vi "Example.vi"() -> ()   [LabVIEW 2019]
uses:
  fd21ea2b-fe82-4c24-8fbe-779a5f18eb94.vi
  193783c4-9c22-43a6-9abe-7ec735545827.vi
  ad1777d4-6ecb-4841-a2c2-9d75e62a62a5.vi
  LV Colormap Names.ctl
panel:
  in  "Stop":bool
  in  "Tab Control":T1(tab)
  in  "Colormap Name (original enum)":T2=enum."turbo"
  in  "Colormap Name (reduced enum)":T3(ring)=enum."inferno"
  in  "Colormap By Name":string="gist_stern"
  in  "Example Data Name":u16(ring)=8 items=["PC Fan"=0, "Noisy Chirps"=1, "TDR 1"=2, "TDR 2"=3, "Liquefaction"=4, "Liquefaction Free"=5, "Aneurysm"=6, "Bat"=7, "RF"=8, "Two Gaussian"=9, "Three Gaussian"=10, "Chirp"=11, "Gaussian Chirp"=12, "Cross Chirp"=13, "Doppler"=14, "HOP"=15, "TF Sine"=16, "Three Tone"=17, "Four Tone"=23, "Blood Flow Doppler (phase a)"=20, "Blood Flow Doppler (phase b)"=21, "Heart sound"=22, "Random Noise"=19]
  out "Signals":waveform(dbl)(graph)={"t0"=timestamp(0 s since 1904-01-01), "dt"=1e-09, "Y"=[]}
  out "Magnitude of Gabor Coefficients":dbl[][](graph)
  # "ex:\nnipy_spectral\ngnuplot\ngist_stern"
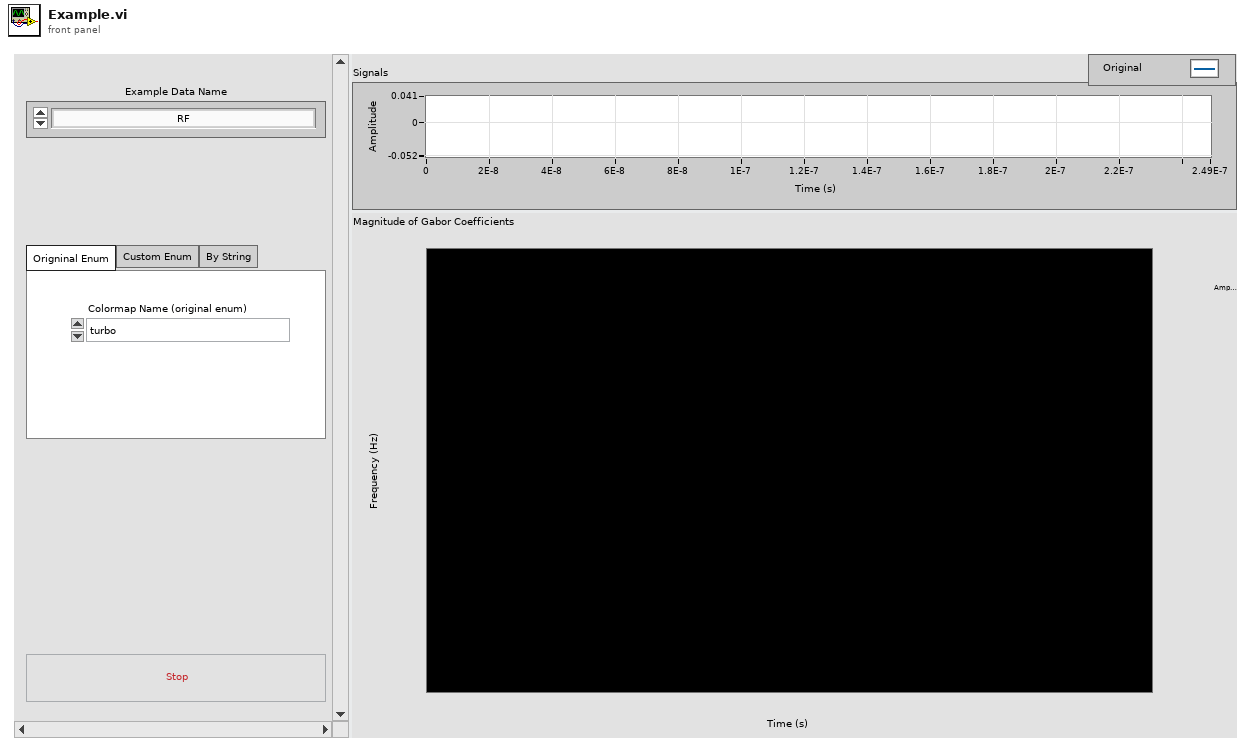
[diagram p1: front panel]
types:
  T1 = enum32{"Origninal Enum", "Custom Enum", "By String"}
  T2 = typedef "LV Colormap Names.ctl" = enum16{"Accent", "Accent_r", "Blues", "Blues_r", "BrBG", "BrBG_r", "BuGn", "BuGn_r", "BuPu", "BuPu_r", "CMRmap", "CMRmap_r", "Dark2", "Dark2_r", "GnBu", "GnBu_r", "Grays", "Grays_r", "Greens", "Greens_r", "Greys", "Greys_r", "OrRd", "OrRd_r", "Oranges", "Oranges_r", "PRGn", "PRGn_r", "Paired", "Paired_r", "Pastel1", "Pastel1_r", "Pastel2", "Pastel2_r", "PiYG", "PiYG_r", "PuBu", "PuBuGn", "PuBuGn_r", "PuBu_r", "PuOr", "PuOr_r", "PuRd", "PuRd_r", "Purples", "Purples_r", "RdBu", "RdBu_r", "RdGy", "RdGy_r", "RdPu", "RdPu_r", "RdYlBu", "RdYlBu_r", "RdYlGn", "RdYlGn_r", "Reds", "Reds_r", "Set1", "Set1_r", "Set2", "Set2_r", "Set3", "Set3_r", "Spectral", "Spectral_r", "Wistia", "Wistia_r", "YlGn", "YlGnBu", "YlGnBu_r", "YlGn_r", "YlOrBr", "YlOrBr_r", "YlOrRd", "YlOrRd_r", "afmhot", "afmhot_r", "autumn", "autumn_r", "berlin", "berlin_r", "binary", "binary_r", "bone", "bone_r", "brg", "brg_r", "bwr", "bwr_r", "cividis", "cividis_r", "cool", "cool_r", "coolwarm", "coolwarm_r", "copper", "copper_r", "cubehelix", "cubehelix_r", "flag", "flag_r", "gist_earth", "gist_earth_r", "gist_gray", "gist_gray_r", "gist_grey", "gist_grey_r", "gist_heat", "gist_heat_r", "gist_ncar", "gist_ncar_r", "gist_rainbow", "gist_rainbow_r", "gist_stern", "gist_stern_r", "gist_yarg", "gist_yarg_r", "gist_yerg", "gist_yerg_r", "gnuplot", "gnuplot2", "gnuplot2_r", "gnuplot_r", "gray", "gray_r", "grey", "grey_r", "hot", "hot_r", "hsv", "hsv_r", "inferno", "inferno_r", "jet", "jet_r", "magma", "magma_r", "managua", "managua_r", "nipy_spectral", "nipy_spectral_r", "ocean", "ocean_r", "pink", "pink_r", "plasma", "plasma_r", "prism", "prism_r", "rainbow", "rainbow_r", "seismic", "seismic_r", "spring", "spring_r", "summer", "summer_r", "tab10", "tab10_r", "tab20", "tab20_r", "tab20b", "tab20b_r", "tab20c", "tab20c_r", "terrain", "terrain_r", "turbo", "turbo_r", "twilight", "twilight_r", "twilight_shifted", "twilight_shifted_r", "vanimo", "vanimo_r", "viridis", "viridis_r", "winter", "winter_r"}
  T3 = enum16{"magma", "inferno", "plasma", "viridis", "cividis", "twilight", "twilight_shifted", "turbo", "berlin", "managua", "vanimo"}
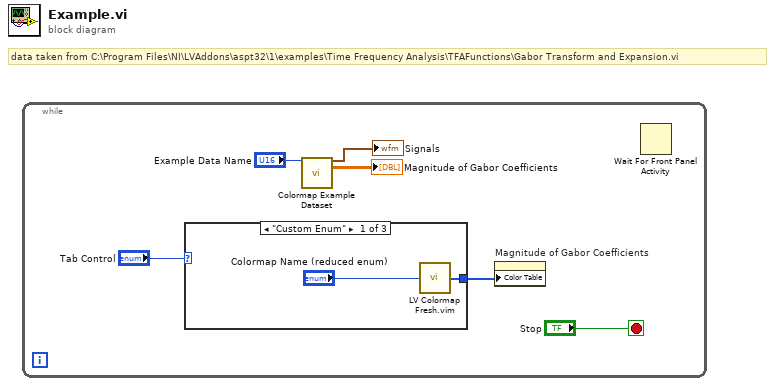
[diagram p0: block diagram]
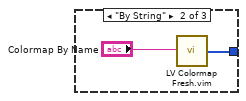
[diagram p2: hidden frame]
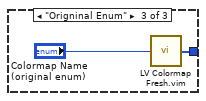
[diagram p3: hidden frame]
diagram:
  # "data taken from C:\\Program Files\\NI\\LVAddons\\aspt32\\1\\examples\\Time Frequency Analysis\\TFAFunctions\\Gabor Transform and Expansion.vi"
  n1 = while {
    stop <- "Stop" stop-if-true
    n2 = case shown="\"Custom Enum\"" "Tab Control" {
      tunnel: [w8 w10 w11] -> w6
      frame "Custom Enum" {
        n3 = call "LV Colormap Fresh.vim"("Colormap Name"="Colormap Name (reduced enum)") -> ("Colormap"=w8:u32[])  [unwired: 14 in]
      }
      frame "By String" {
        n4 = call "LV Colormap Fresh.vim"("Colormap Name"="Colormap By Name") -> ("Colormap"=w10:u32[])  [unwired: 14 in]
      }
      frame "Origninal Enum" {
        n5 = call "LV Colormap Fresh.vim"("Colormap Name"="Colormap Name (original enum)") -> ("Colormap"=w11:u32[])  [unwired: 14 in]
      }
    }
    n6 = call "Colormap Example Dataset.vi"("Example Data Name"="Example Data Name") -> ("Waveform"=→"Signals":waveform(dbl), "TF coefficients indicator"=→"Magnitude of Gabor Coefficients":dbl[][])  [unwired: 13 in]
    n7 = property on="Magnitude of Gabor Coefficients" class="IntGraph (strict)"("Color Table"=w6) -> ()  [unwired: 2 in, 2 out]
    n8 = Wait For Front Panel Activity() -> ()  [unwired: 3 in, 1 out]
  }
